vi "LVClass_Camera ctor.vi"(0 "Camera (const)":refnum<class "Camera.lvclass">, 5 "Configuration file path":path, 11 "error in (no error)":errorcluster) -> (4 "Camera (new)":refnum<class "Camera.lvclass">, 15 "error out":errorcluster)   [LabVIEW 2020, in "Camera.lvclass"]
doc: "Camera constructor.\n\n<B>CameraIn</B> : Constant Pointer to Camera object, Camera connection is automatically\n established to the device. (no neeed to use Imop_Camera_Connect)\n<B>CameraOut</B> : Constant Pointer to Camera object, Camera connection is automatically\n established to the device. (no neeed to use Imop_Camera_Connect)\n<B>config_file_path</B> : Absolute path to Haso or Camera configuration file."
uses:
  Camera.lvclass
  Handle creation.ctl
  Camera.lvclass/Camera.ctl
  CameraSet.lvclass
  Image.lvclass
  Data alignment enum.ctl
  CameraAcquisitionState.ctl
  LVClass_CameraSet Read CameraParameters.vi
  LVClass_CameraSet Read AllValueSetAndGet.vi
  LVClass_CameraSet Read AllValueGet.vi
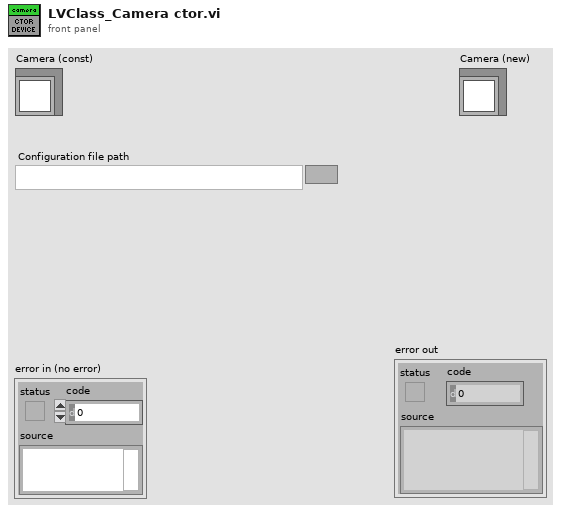
[diagram p1: front panel]
types:
  T1 = typedef "Handle creation.ctl" = enum16{"By ctor", "By write function"}
  T2 = typedef "Data alignment enum.ctl" = enum16{"8", "16", "32"}
  T3 = typedef "CameraAcquisitionState.ctl" = enum16{"Stop", "Live"}
  T4 = typedef "ParameterID.ctl" = cluster{"Name":string, "ConnectionParameter?":bool, "Type":T5, "Authorization":T6, "OnFlyAuthorization":T7, "StringValue":string, "Value":dbl, "Min":dbl, "Max":dbl, "BooleanValue":bool, "StringParameterList":string[]}
  T5 = typedef "CameraParameters_Type.ctl" = enum16{"Integer", "Real", "String", "Boolean"}
  T6 = typedef "CameraParameters_Authorization.ctl" = enum16{"Disable", "Gettable", "Settable - Gettable"}
  T7 = typedef "CameraParameters_OnFlyAuthorization.ctl" = enum16{"None", "Gettable", "Settable", "Settable - Gettable"}
  T8 = typedef "CameraParametersSetup.ctl" = cluster{"Name":string, "Type":T5, "Value":dbl, "BooleanValue":bool, "StringValue":string, "ConnectionParameter":bool}
  T9 = typedef "CameraSpecifications.ctl" = cluster{"Grabber name":string, "Camera name":string, "Camera sn":string, "Pixels_um":T10, "Maximum level":u32, "Data alignment":T2, "Is signed":bool, "Acquisition start":T11, "Acquisition length":T11, "MaxFrameRate_Hz":sgl, "Chip type":enum16{"Progressive scan", "Frame transfert"}}
  T10 = typedef "General dimensions definition.ctl" = cluster{"Size":T11, "Step":T12}
  T11 = typedef "Point2D.ctl" = cluster{"X":u32, "Y":u32}
  T12 = typedef "Point2Df.ctl" = cluster{"X":sgl, "Y":sgl}
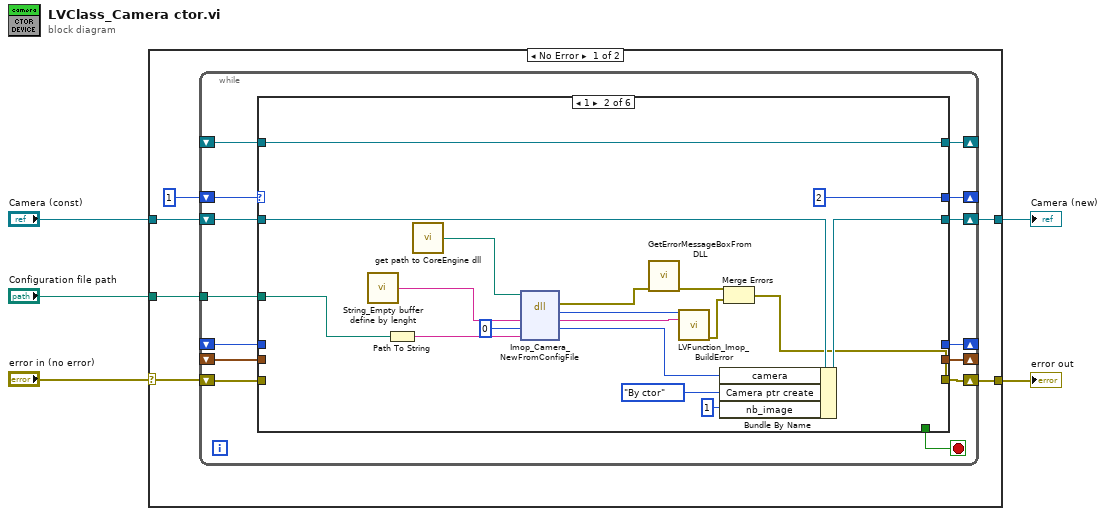
[diagram p0: block diagram]
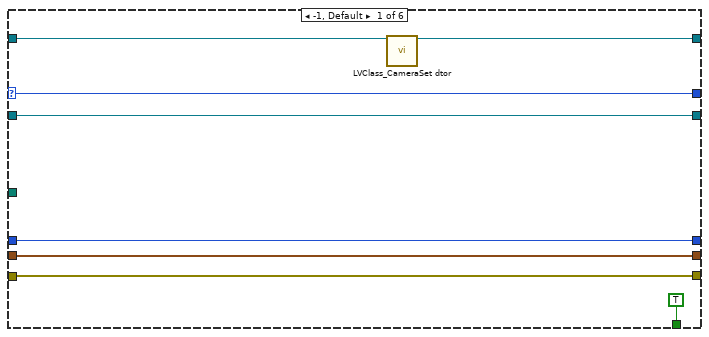
[diagram p2: hidden frame]
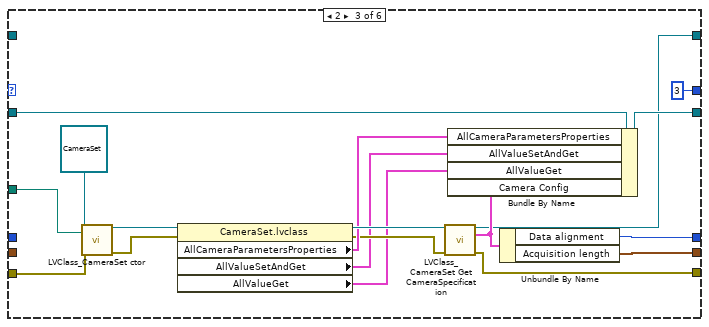
[diagram p3: hidden frame]
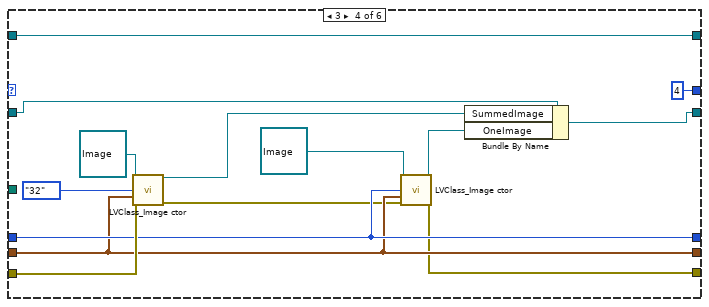
[diagram p4: hidden frame]
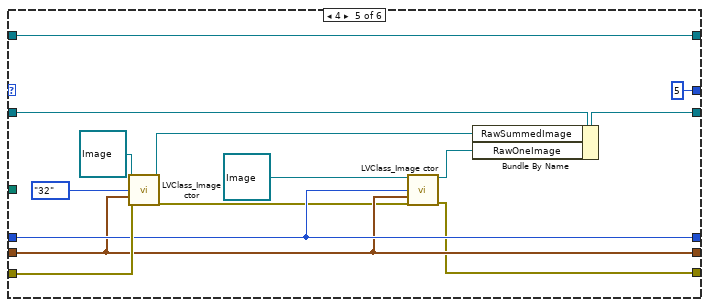
[diagram p5: hidden frame]
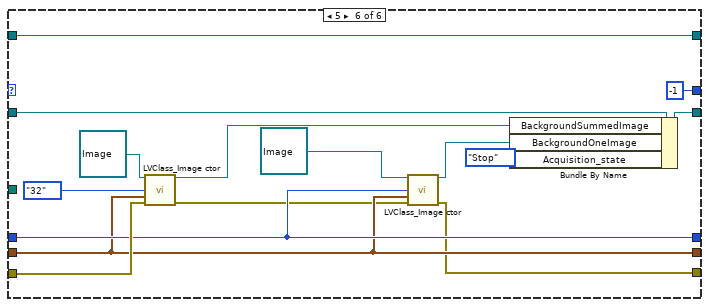
[diagram p6: hidden frame]
diagram:
  n1 = case shown="No Error" "error in (no error)" {
    selector: "error in (no error)" -> [w7 w114]
    tunnel: [w6 w114] -> w4
    tunnel: [w10 w113] -> w2
    tunnel: "Camera (const)" -> [w11 w113]
    tunnel: "Configuration file path" -> [w8 _]
    frame No Error {
      n2 = while {
        shift-right: [w23] -> _
        shift-left: 1 -> [w22]
        tunnel: w8 -> [w21]
        shift-right: [w20] -> w6
        shift-left: w7 -> [w19]
        shift-right: [w17] -> _
        shift-left: _ -> [w15]
        shift-right: [w18] -> _
        shift-left: _ -> [w16]
        shift-right: [w24] -> w10
        shift-left: w11 -> [w25]
        shift-right: [w13] -> _
        shift-left: _ -> [w12]
        stop <- w14 stop-if-true
        n3 = case shown="1" w22 {
          selector: w22 -> [w32 _ _ _ _ _]
          tunnel: [w31 w35 w65 w73 w87 w102] -> w20
          tunnel: w25 -> [w28 w46 w62 w81 w95 w110]
          tunnel: [w28 w45 w61 w80 w94 w109] -> w24
          tunnel: [w32 2 3 4 5 -1] -> w23
          tunnel: w21 -> [_ w40 w68 _ _ _]
          tunnel: w19 -> [w31 _ w67 w82 w96 w111]
          tunnel: [w29 _ w63 w77 w91 w106] -> w18
          tunnel: [w30 _ w66 w76 w90 w105] -> w17
          tunnel: w16 -> [w29 _ _ w77 w91 w106]
          tunnel: w15 -> [w30 _ _ w76 w90 w105]
          tunnel: [TRUE _ _ _ _ _] -> w14
          tunnel: [w26 w38 w55 w71 w85 w100] -> w13
          tunnel: w12 -> [w27 w38 _ w71 w85 w100]
          frame -1, Default {
            n4 = call "LVClass_CameraSet dtor.vi"("CameraSet in"=w27) -> ("CameraSet out"=w26:refnum<class "CameraSet.lvclass">)  [unwired: 13 in, 1 out]
          }
          frame 1 {
            n5 = call "String_Empty buffer define by lenght.vi"() -> ("Empty buffer"=w44:string)  [unwired: 1 in]
            n6 = Path To String(path=w40) -> (string=w39:string)
            n7 = call "get path to CoreEngine dll.vi"() -> ("path to c_interface_vc100.dll"=w43:path)  [unwired: 12 in, 3 out]
            n8 = dll-call lib="D:/soft/HASO_v3/SVN_trunk/ImOpCoreEngine4_LV2011/DLLs/c_interface_vc100.dll" fn="Imop_Camera_NewFromConfigFile"(path in=w43, "message"=w44, "objet"=0, "chemin_config"=w39) -> (error out=w42:errorcluster, "return type"=w49:i32, "message"=w48:string, "objet"=w47:i64)  [unwired: 3 in, 1 out]
            n9 = call "GetErrorMessageBoxFromDLL.vi"("error IN"=w42) -> ("error OUT"=w37:errorcluster)  [unwired: 10 in]
            n10 = call "LVFunction_Imop_BuildError.vi"("code"=w49, "String to Prepend to source (\"\")"=w48) -> ("error out"=w36:errorcluster)  [unwired: 13 in]
            n11 = Bundle By Name(cluster=w46, "camera"=w47, "Camera ptr create"=Handle_creation."By ctor" ("Haso ptr create"), "nb_image"=u32 1) -> (w45:refnum<class "Camera.lvclass">)
            n12 = Merge Errors(w37, w36) -> (w35:errorcluster)
          }
          frame 2 {
            n13 = call "LVClass_CameraSet ctor.vi"("CameraSet (const)"=refnum<class "CameraSet.lvclass"> refnum ("CameraSet.lvclass"), "Configuration file path"=w68, "error in (no error)"=w67) -> ("CameraSet (new)"=w53:refnum<class "CameraSet.lvclass">, "error out"=w52:errorcluster)  [unwired: 11 in]
            n14 = property class="CameraSet.lvclass"(reference=w53, error in=w52) -> (reference out=w60:refnum<class "CameraSet.lvclass">, error out=w58:errorcluster, "AllCameraParametersProperties"=w59:T4[], "AllValueSetAndGet"=w57:T8[], "AllValueGet"=w54:T8[])
            n15 = call "LVClass_CameraSet Get CameraSpecification.vi"("CameraSet in"=w60, "error in (no error)"=w58) -> ("CameraSet out"=w55:refnum<class "CameraSet.lvclass">, "Camera Config"=w56:T9, "error out"=w65:errorcluster)  [unwired: 11 in]
            n16 = Bundle By Name(cluster=w62, "AllCameraParametersProperties"=w59, "AllValueSetAndGet"=w57, "AllValueGet"=w54, "Camera Config"=w56) -> (w61:refnum<class "Camera.lvclass">)
            n17 = Unbundle By Name(w56) -> ("Data alignment"=w63:T2, "Acquisition length"=w66:T11)
          }
          frame 3 {
            n18 = call "LVClass_Image ctor.vi"("Image (const)"=refnum<class "Image.lvclass"> refnum ("Image in"), "Data alignment"=Data_alignment_enum."32", "Size"=w76, "error in (no error)"=w82) -> ("Image (new)"=w79:refnum<class "Image.lvclass">, "error out"=w74:errorcluster)  [unwired: 10 in]
            n19 = call "LVClass_Image ctor.vi"("Image (const)"=refnum<class "Image.lvclass"> refnum ("Image in"), "Data alignment"=w77, "Size"=w76, "error in (no error)"=w74) -> ("Image (new)"=w75:refnum<class "Image.lvclass">, "error out"=w73:errorcluster)  [unwired: 10 in]
            n20 = Bundle By Name(cluster=w81, "SummedImage"=w79, "OneImage"=w75) -> (w80:refnum<class "Camera.lvclass">)
          }
          frame 4 {
            n21 = call "LVClass_Image ctor.vi"("Image (const)"=refnum<class "Image.lvclass"> refnum ("Image in"), "Data alignment"=Data_alignment_enum."32", "Size"=w90, "error in (no error)"=w96) -> ("Image (new)"=w93:refnum<class "Image.lvclass">, "error out"=w88:errorcluster)  [unwired: 10 in]
            n22 = call "LVClass_Image ctor.vi"("Image (const)"=refnum<class "Image.lvclass"> refnum ("Image in"), "Data alignment"=w91, "Size"=w90, "error in (no error)"=w88) -> ("Image (new)"=w89:refnum<class "Image.lvclass">, "error out"=w87:errorcluster)  [unwired: 10 in]
            n23 = Bundle By Name(cluster=w95, "RawSummedImage"=w93, "RawOneImage"=w89) -> (w94:refnum<class "Camera.lvclass">)
          }
          frame 5 {
            n24 = call "LVClass_Image ctor.vi"("Image (const)"=refnum<class "Image.lvclass"> refnum ("Image in"), "Data alignment"=Data_alignment_enum."32", "Size"=w105, "error in (no error)"=w111) -> ("Image (new)"=w108:refnum<class "Image.lvclass">, "error out"=w103:errorcluster)  [unwired: 10 in]
            n25 = call "LVClass_Image ctor.vi"("Image (const)"=refnum<class "Image.lvclass"> refnum ("Image in"), "Data alignment"=w106, "Size"=w105, "error in (no error)"=w103) -> ("Image (new)"=w104:refnum<class "Image.lvclass">, "error out"=w102:errorcluster)  [unwired: 10 in]
            n26 = Bundle By Name(cluster=w110, "BackgroundSummedImage"=w108, "BackgroundOneImage"=w104, "Acquisition_state"=CameraAcquisitionState."Stop") -> (w109:refnum<class "Camera.lvclass">)
          }
        }
      }
    }
    frame Error {
    }
  }
  "error out" <- w4
  "Camera (new)" <- w2
